vi "speak.vi"(8 "error in (no error)":errorcluster, 11 "BabyHuman in":refnum<class "BabyHuman.lvclass">) -> (0 "error out":errorcluster, 2 "message":string, 3 "BabyHuman out":refnum<class "BabyHuman.lvclass">)   [LabVIEW 2017, in "BabyHuman.lvclass"]
uses:
  BabyHuman.lvclass
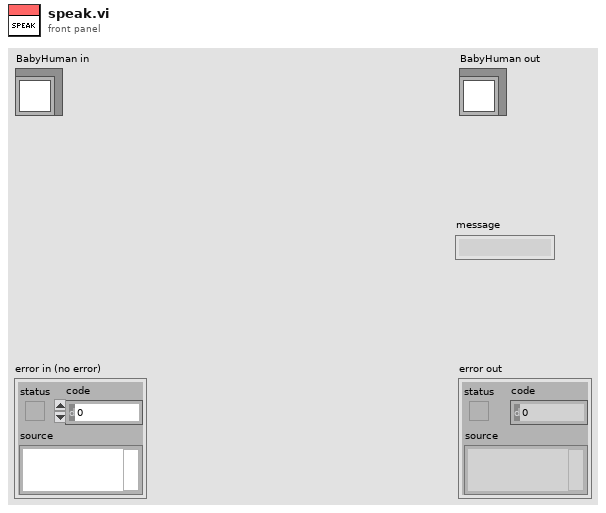
[diagram p1: front panel]
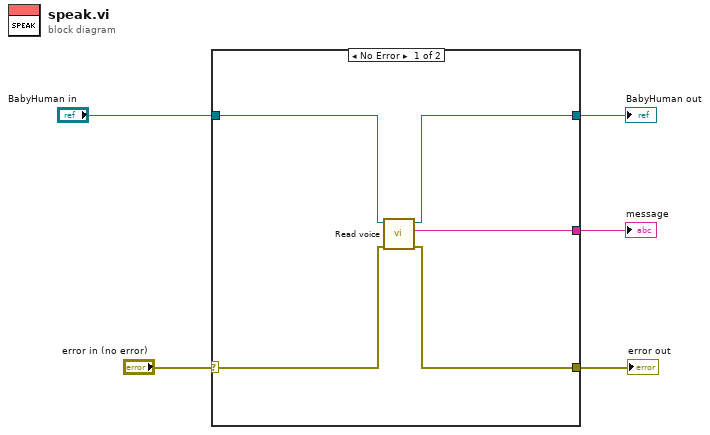
[diagram p0: block diagram]
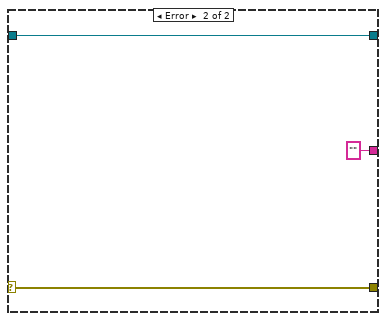
[diagram p2: hidden frame]
diagram:
  n1 = case shown="No Error" "error in (no error)" {
    selector: "error in (no error)" -> [w8 w11]
    tunnel: [w7 w11] -> w4
    tunnel: [w9 w13] -> w3
    tunnel: "BabyHuman in" -> [w10 w13]
    tunnel: [w6 "" ("voice")] -> w1
    frame No Error {
      n2 = call-dynamic "Read voice.vi"("error in (no error)"=w8, "BabyHuman in"=w10) -> ("error out"=w7:errorcluster, "voice"=w6:string, "BabyHuman out"=w9:refnum<class "BabyHuman.lvclass">)  [unwired: 7 in]
    }
    frame Error {
    }
  }
  "error out" <- w4
  "BabyHuman out" <- w3
  "message" <- w1
